vi "Write Setpoint.vi"(8 "error in":errorcluster, 10 "SP":sgl, 11 "TE Cooler in":refnum<class "TE Cooler.lvclass">) -> (0 "error out":errorcluster, 3 "TE Cooler out":refnum<class "TE Cooler.lvclass">)   [LabVIEW 2018, in "TE Cooler.lvlib" / "TE Cooler.lvclass"]
doc: "Write the setpoint of the controller in whatever units are specified."
uses:
  TE Cooler.lvclass
  Controls/Command.ctl
  TE Cooler.lvclass/TE Cooler.ctl
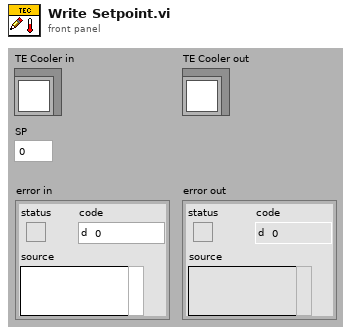
[diagram p1: front panel]
types:
  T1 = typedef "TE Cooler.lvlib/TE Cooler.lvclass/Command.ctl" = enum16{"INPUT1", "DESIRED CONTROL VALUE", "POWER OUTPUT", "ALARM STATUS", "INPUT 2", "OUTPUT CURRENT COUNTS", "ALARM TYPE", "SET TYPE DEFINE", "SENSOR TYPE", "CONTROL TYPE", "CONTROL OUTPUT POLARITY", "POWER ON/OFF", "OUTPUT SHUTDOWN IF ALARM", "FIXED DESIRED CONTROL SETTING", "PROPORTIONAL BANDWIDTH", "INTEGRAL GAIN", "DERIVATIVE GAIN", "LOW EXTERNAL SET RANGE", "HIGH EXTERNAL SET RANGE", "ALARM DEADBAND", "HIGH ALARM SETTING", "LOW ALARM SETTING", "CONTROL DEADBAND SETTING", "INPUT1 OFFSET", "INPUT2 OFFSET", "HEAT MULTIPLIER", "COOL MULTIPLIER", "OVER CURRENT COUNT COMPARE VALUE", "ALARM LATCH ENABLE", "NOT USED", "ALARM LATCH RESET", "CHOOSE SENSOR FOR ALARM FUNCTION", "CHOOSE TEMPERATURE WORKING UNITS", "EEPROM WRITE ENABLE", "OVER CURRENT CONTINUOUS", "OVER CURRENT RESTART ATTEMPTS", "JP3 DISPLAY ENABLE"}
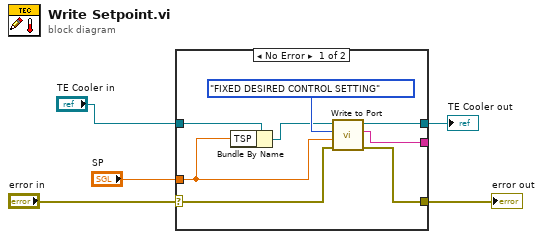
[diagram p0: block diagram]
diagram:
  n1 = case shown="No Error" "error in" {
    selector: "error in" -> [w11 w15]
    tunnel: [w10 w15] -> w4
    tunnel: [w13 w14] -> w2
    tunnel: "TE Cooler in" -> [w9 w14]
    tunnel: "SP" -> [w7 _]
    tunnel: [w6 _] -> _
    frame No Error {
      n2 = Bundle By Name(cluster=w9, "TSP"=w7) -> (w8:refnum<class "TE Cooler.lvclass">)
      n3 = call "Write to Port.vi"("error in"=w11, "Input Value"=w7, "TEC Cmd"=Command."FIXED DESIRED CONTROL SETTING", "TE Cooler in"=w8) -> ("error out"=w10:errorcluster, "String"=w6:string, "TE Cooler out"=w13:refnum<class "TE Cooler.lvclass">)  [unwired: 5 in]
    }
    frame Error {
    }
  }
  "error out" <- w4
  "TE Cooler out" <- w2
